vi "Lab Send Mail Test.vi"(0 "TO:":string, 1 "subject":string, 2 "Info":string, 5 "from":string, 7 "out going server":string, 9 "message":string, 11 "username":string, 12 "password":string, 13 "Attachements":path[](array[path])) -> (15 "error out":errorcluster)   [LabVIEW 2017]
uses:
  <vilib>/Utility/error.llb/DialogType.ctl
  <vilib>/Utility/SMTP/NI_SMTPEmail.lvlib
panel:
  out "message 2":string=" INSTRUCTIONS:\r\rNormal Use:  When using subVIs that incorporate the error in/error out (or error I/O) structure, place this handler where you want to inform the user of an error, typically at the end of the I/O data path, as the last action of the program.  If the error in error? is ERROR, the handler creates a message describing the error and its source.  If the type of dialog = 1 (default), the message is displayed to the user, who can only acknowedge it.  If the type = 2, the user can acknowledge the message or abort execution; aborting a program with active I/O is not recommended.  If the type = 0, no message is displayed; this is used to process the error programmatically, and the error out cluster elements are wired to individual terminals for that reason.  \r\rOther Use:\n\r\nlocal testing.  To test the error code of a subVI or function that does not have the error I/O structure, you can wire its error code and a source string to the local error code and error source inputs.  If error in error? indicates no error and error code is not equal to 0, the local code and source are substituted for the error in values, and error? is set TRUE (ERROR)."
  in  "Tab Control":enum32{"Page 1", "Page 2"}(tab)
  in  "Mail To:":string[](array[string])
  # "SENDING MAIL"
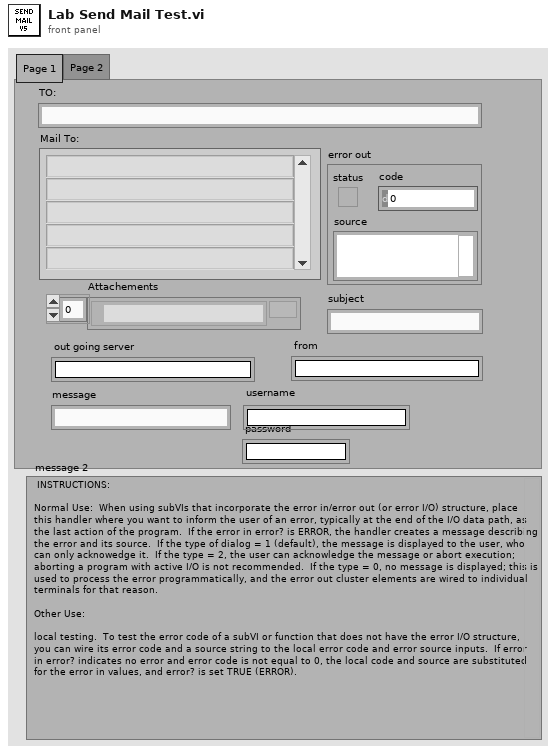
[diagram p1: front panel]
types:
  T1 = typedef "DialogType.ctl" = u16
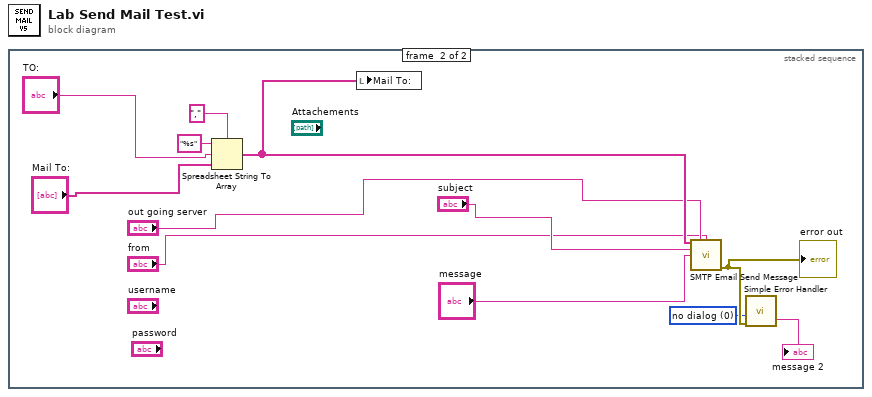
[diagram p0: block diagram]
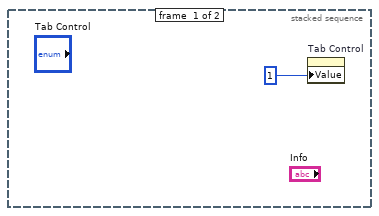
[diagram p2: hidden frame]
diagram:
  n1 = stacked-sequence {
    frame #0 {
      n2 = property on="Tab Control" class="TabCtl (strict)"("Value"=1) -> ()  [unwired: 2 in, 2 out]
    }
    frame #1 {
      w3 = T1 0 items=["no dialog", "OK message", "continue or stop message", "OK message + warnings", "continue/stop + warnings"] ("type of dialog (OK msg:1)")
      n3 = Spreadsheet String To Array(delimiter (Tab)=",", format string="%s", spreadsheet string="TO:", array type (2D Dbl)="Mail To:") -> (array=w8:string[])
      n4 = local write "Mail To:"(w8) -> ()
      n5 = call <vilib>:"SMTP Email Send Message.vi"("recipients"=w8, "mail server"="out going server", "return address"="from", "subject ([No Subject])"="subject", "message"="message") -> ("error out"=w4:errorcluster)  [unwired: 9 in, 1 out]
      "error out" <- w4
      n6 = call <vilib>:"Simple Error Handler.vi"("type of dialog (OK msg:1)"=w3, "error in (no error)"=w4) -> ("message"=→"message 2":string)  [unwired: 3 in, 4 out]
    }
  }
